vi "Impedance tube v0.4_Signal_FFT.vi"() -> ()   [LabVIEW 2021]
uses:
  <vilib>/Analysis/2dsp.llb/Real FFT.vi
  <vilib>/express/express analysis/Spectral/Block/exnSpectralBlock spectral measurements RMS poly.vi
  <vilib>/express/express analysis/Spectral/Block/exnSpectralBlock spectral measurements RMS DDT.vi
  <vilib>/express/express arith-compare/Formula/XNode/ExpressFormulaBlockNode.xnode
  <vilib>/express/express analysis/Spectral/XNode/ExpressSpectralMeasurementsBlockNode.xnode
  <vilib>/Analysis/NI_AALPro.lvlib
panel:
  out "Waveform Graph 3":dynamicdata(graph)
  out "Waveform Graph":dynamicdata(graph)
  out "Numeric":dbl
  out "x + iy 3":cdb
  out "x + iy 2":cdb
  out "x + iy":cdb
  out "Result 2":csg
  out "Result":csg
  out "probe 3":dynamicdata(graph)
  out "probe 2":dynamicdata(graph)
  out "Transfer function":dynamicdata(graph)
  out "Waveform Graph 2":dynamicdata(graph)
  out "probe 1":dynamicdata(graph)
  out "Reflection coefficient":dynamicdata(graph)
  out "FFT {2}":cdb[](array[numeric])
  out "MIC 2":dynamicdata(graph)
  out "FFT2":dynamicdata(graph)
  in  "FFT size 2":i32=-1
  out "MIC 2":dbl
  out "FFT1":dynamicdata(graph)
  out "MIC 1":dynamicdata(graph)
  in  "FFT size":i32=-1
  out "MIC 1":dbl
  in  "stop (F)":bool
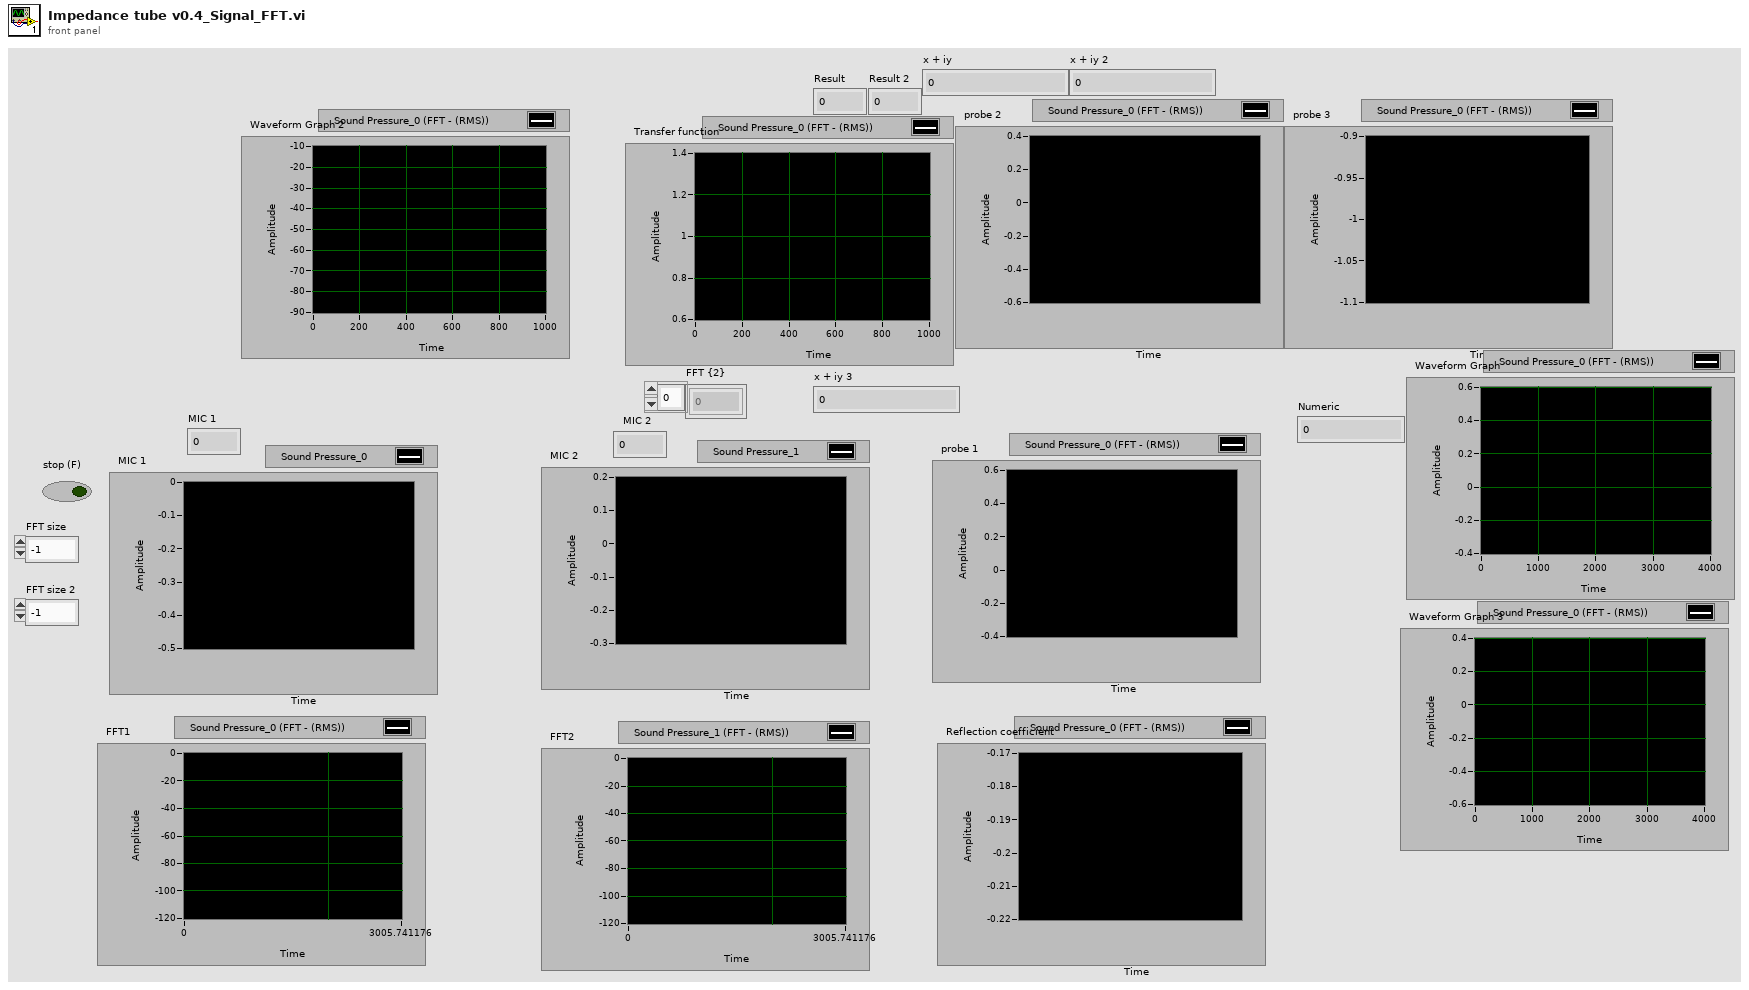
[diagram p1: front panel]
types:
  T1 = cluster{"averaging mode":u16, "weighting mode":u16, "number of averages":u32}
  T2 = cluster{"dB On (F)":bool, "unwrap phase (F)":bool, "convert to degree (F)":bool}
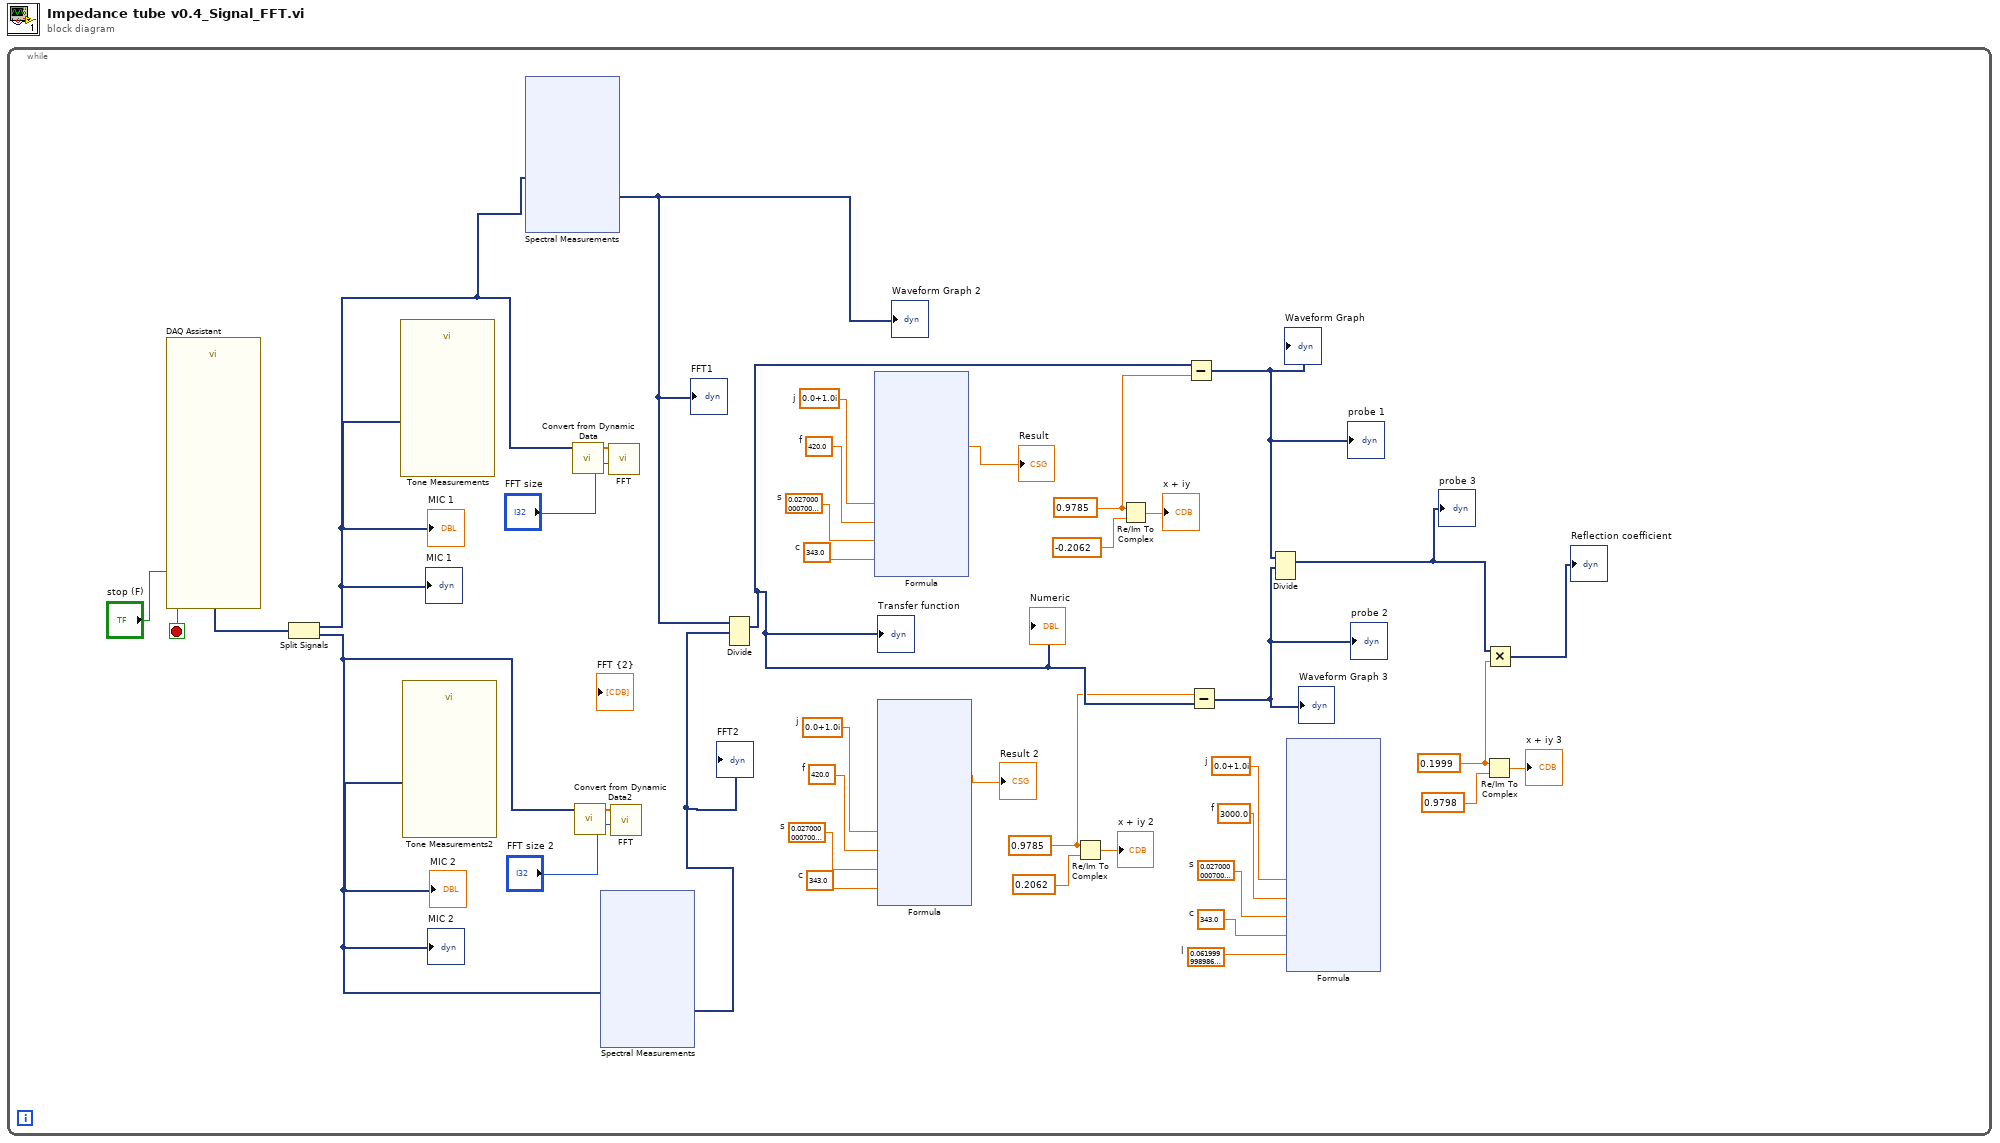
[diagram p0: block diagram]
diagram:
  n1 = while {
    stop <- w39 stop-if-true
    w1 = 0.1999 ("x")
    w3 = 0.9785 ("x")
    w2 = 0.9785 ("x")
    w19 = sgl 0.062  # l
    w22 = sgl 3000.0  # f
    w21 = sgl 0.027  # s
    w20 = sgl 343.0  # c
    w23 = csg 0.0+1.0i  # j
    w27 = sgl 420.0  # f
    w26 = sgl 0.027  # s
    w25 = sgl 343.0  # c
    w28 = csg 0.0+1.0i  # j
    w32 = sgl 420.0  # f
    w31 = sgl 0.027  # s
    w30 = sgl 343.0  # c
    w33 = csg 0.0+1.0i  # j
    n2 = call "DAQ Assistant"("stop (F)"="stop (F)") -> ("data"=w36:dynamicdata, "stopped"=w39:bool)  [unwired: 15 in, 2 out]
    n3 = Split Signals(w36) -> (w17:dynamicdata, w16:dynamicdata)  [unwired: 2 in]
    "MIC 1" <- w17
    "MIC 1" <- w17
    "MIC 2" <- w16
    "MIC 2" <- w16
    n4 = call "Tone Measurements"("Signals"=w17) -> ()  [unwired: 8 in, 3 out]
    n5 = call "Tone Measurements2"("Signals"=w16) -> ()  [unwired: 8 in, 3 out]
    n6 = xnode "Spectral Measurements"("Signals"=w17) -> ("FFT - (RMS)"=w13:dynamicdata)  [unwired: 1 in, 2 out]
    "FFT1" <- w13
    "Waveform Graph 2" <- w13
    n7 = call "Convert from Dynamic Data"("Dynamic Data Type"=w17) -> ("Array"=w37:dbl[])  [unwired: 3 in]
    n8 = call "Convert from Dynamic Data2"("Dynamic Data Type"=w16) -> ("Array"=w34:dbl[])  [unwired: 3 in]
    n9 = xnode "Spectral Measurements"("Signals"=w16) -> ("FFT - (RMS)"=w15:dynamicdata)  [unwired: 1 in, 2 out]
    "FFT2" <- w15
    n10 = call-poly <vilib>:"FFT.vi"("FFT size"="FFT size", "X"=w37) -> ()  [unwired: 8 in, 2 out]
    n11 = call-poly <vilib>:"FFT.vi"("FFT size"="FFT size 2", "X"=w34) -> ()  [unwired: 8 in, 2 out]
    n12 = Divide(1:w15, 2:w13) -> (0:w14:dynamicdata)  [unwired: 1 in, 1 out]
    "Transfer function" <- w14
    "Numeric" <- w14
    n13 = xnode "Formula"("j"=w33, "f"=w32, "s"=w31, "c"=w30) -> ("Result"=→"Result":dbl)  [unwired: 1 in, 1 out]
    n14 = xnode "Formula"("j"=w28, "f"=w27, "s"=w26, "c"=w25) -> ("Result"=→"Result 2":dbl)  [unwired: 1 in, 1 out]
    n15 = Re/Im To Complex(1:0.2062 ("y"), 2:w3) -> (0:→"x + iy 2":cdb)
    n16 = Re/Im To Complex(1:-0.2062 ("y"), 2:w2) -> (0:→"x + iy":cdb)
    n17 = Subtract(x=w14, y=w2) -> (x-y=w12:dynamicdata)
    "probe 1" <- w12
    "Waveform Graph" <- w12
    n18 = Subtract(x=w3, y=w14) -> (x-y=w11:dynamicdata)
    "probe 2" <- w11
    "Waveform Graph 3" <- w11
    n19 = Divide(1:w11, 2:w12) -> (0:w10:dynamicdata)  [unwired: 1 in, 1 out]
    "probe 3" <- w10
    n20 = xnode "Formula"("j"=w23, "f"=w22, "s"=w21, "c"=w20, "l"=w19) -> ()  [unwired: 1 in, 2 out]
    n21 = Re/Im To Complex(1:0.9798 ("y"), 2:w1) -> (0:→"x + iy 3":cdb)
    n22 = Multiply(x=w10, y=w1) -> (x*y=→"Reflection coefficient":dynamicdata)
  }
